vi "Initialize Hardware References.vi"(8 "error in (no error)":errorcluster, 10 "Hardware Config \nCluster":T1 {"Unit" items=["Volts", "From Custom Scale"]}, 11 "HW Refnum":string) -> (0 "error out":errorcluster, 2 "Hardware Config Out":T1 {"Unit" items=["Volts", "From Custom Scale"]}, 3 "HW Refnum":string)   [LabVIEW 2020, in "Acquisition.lvlib"]
doc: "Initialize the hardware references.\n_____\nBased on DQMH Project Template 6.0.0.91."
uses:
  Acquisition.lvlib
  Settings Editor/DAQmx Config--cluster.ctl
  Settings Editor/Settings Editor.lvlib
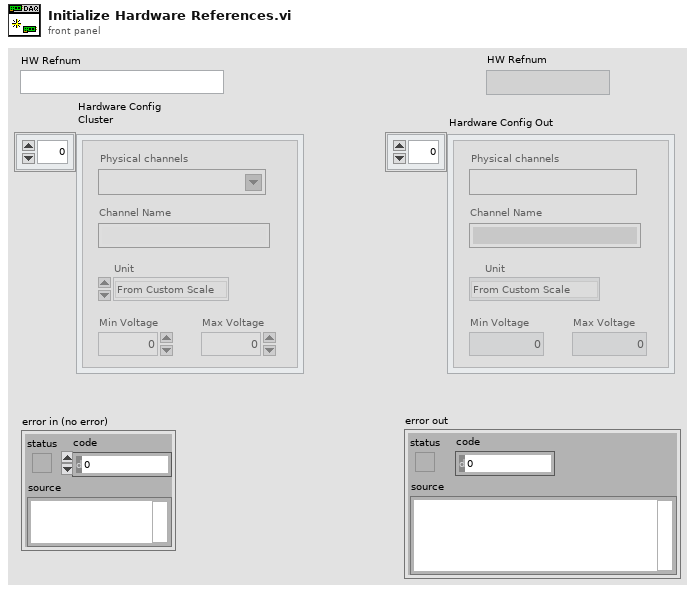
[diagram p1: front panel]
types:
  T1 = typedef "Settings Editor.lvlib/DAQmx Config--cluster.ctl" = cluster{"Physical channels":tag, "Channel Name":string, "Unit":i32, "Min Voltage":dbl, "Max Voltage":dbl}[]
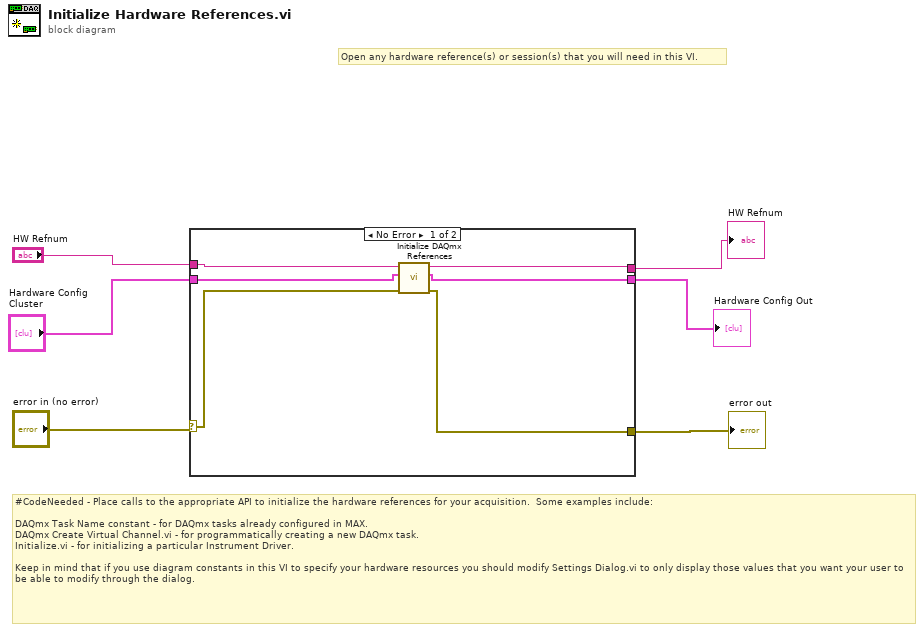
[diagram p0: block diagram]
diagram:
  # "Open any hardware reference(s) or session(s) that you will need in this VI."
  # "#CodeNeeded - Place calls to the appropriate API to initialize the hardware references for your acquisition.  Some examples include:\n\nDAQmx Task Name constant - for DAQmx tasks already configured in MAX.\nDAQmx Create Virtual Channel.vi - for programmatically creating a new DAQmx task.\nInitialize.vi - for initializing a particular Instrument Driver.\n\nKeep in mind that if you use diagram constants in this VI to specify your hardware resources you should modify Settings Dialog.vi to only display those values that you want your user to be able to modify through the dialog."
  n1 = case shown="No Error" "error in (no error)" {
    selector: "error in (no error)" -> [w10 w15]
    tunnel: [w11 w15] -> w5
    tunnel: [w12 w14] -> w3
    tunnel: "Hardware Config \nCluster" -> [w8 w13]
    tunnel: "HW Refnum" -> [w9 w14]
    tunnel: [w7 w13] -> w2
    frame No Error {
      n2 = call "Initialize DAQmx References.vi"("error in (no error)"=w10, "Hardware Config Cluster"=w8, "Task Name"=w9) -> ("error out"=w11:errorcluster, "Hardware Config Cluster Out"=w7:T1, "HW Refnum Out"=w12:string)  [unwired: 6 in]
    }
    frame Error {
    }
  }
  "error out" <- w5
  "HW Refnum" <- w3
  "Hardware Config Out" <- w2
